vi "TDT-Get Target (1D DBL).vi"(0 "Data":T1={"TTankX"=refnum, "TDevAccX"=refnum, "LastTime"=0.0, "error"={"status"=FALSE, "code"=0, "source"=""}, "Block Name"="", "Circuit Tag"="", "Tank Name"="", "NumTicks"=0, "LastTick"=0.0, "Idle?"=FALSE, "Wait (ms)"=1000, "LastArtf"=0.0, "LastTosc"=0.0}, 7 "Target":string, 11 "error in (no error)":errorcluster) -> (8 "Val":dbl[](array[numeric]), 15 "error out":errorcluster)   [LabVIEW 2015]
uses:
  TDT Interface Data.ctl
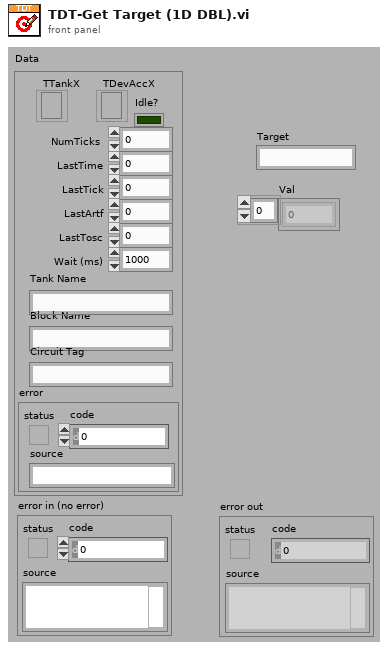
[diagram p1: front panel]
types:
  T1 = typedef "TDT Interface Data.ctl" = cluster{"TTankX":refnum<k7>, "TDevAccX":refnum<k7>, "LastTime":dbl, "error":errorcluster, "Block Name":string, "Circuit Tag":string, "Tank Name":string, "NumTicks":i32, "LastTick":dbl, "Idle?":bool, "Wait (ms)":u32, "LastArtf":dbl, "LastTosc":dbl}
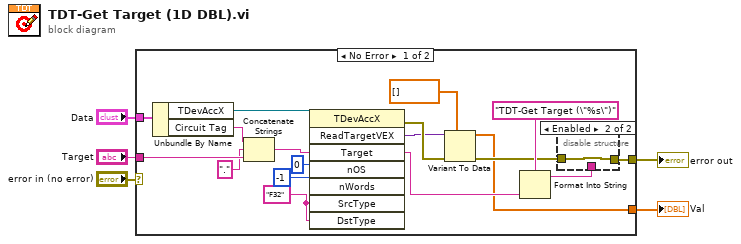
[diagram p0: block diagram]
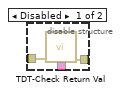
[diagram p2: hidden frame]
diagram:
  n1 = case shown="No Error" "error in (no error)" {
    selector: "error in (no error)" -> [_ w28]
    tunnel: [w17 w28] -> w4
    tunnel: "Data" -> [w22 _]
    tunnel: "Target" -> [w20 _]
    tunnel: [w8 _] -> w1
    frame No Error {
      w7 = "F32" ("DstType")
      n2 = Unbundle By Name(w22) -> ("TDevAccX"=w23:refnum<k7>, "Circuit Tag"=w21:string)
      n3 = Concatenate Strings(w21, "." ("string"), w20) -> (w18:string)
      n4 = invoke class="TDevAccX" method="ReadTargetVEX"(reference=w23, "Target"=w18, "nOS"=0, "nWords"=-1, "SrcType"=w7, "DstType"=w7) -> (error out=w12:errorcluster, "ReadTargetVEX"=w11:variant, "Target"=w14:string)  [unwired: 2 in, 5 out]
      n5 = Variant To Data(error in=w12, type=dbl[] [] ("Val"), Variant=w11) -> (data=w8:dbl[], error out=w10:errorcluster)
      n6 = Format Into String(format string="TDT-Get Target (\"%s\")" ("source"), w14) -> (resulting string=w13:string)  [unwired: 2 in, 1 out]
      n7 = disable-structure shown="Enabled" {
        disable-tunnel: [w26 w27] -> w17
        disable-tunnel: w13 -> [w25 _]
        disable-tunnel: w10 -> [w24 w27]
        frame Disabled {
          n8 = call "TDT-Check Return Val.vi"("error in (no error)"=w24, "source"=w25) -> ("error out"=w26:errorcluster)  [unwired: 13 in]
        }
        frame Enabled {
        }
      }
    }
    frame Error {
    }
  }
  "error out" <- w4
  "Val" <- w1
